vi "Dc_transparency_test_2.vi"() -> ()   [LabVIEW 2013]
uses:
  <vilib>/DAQmx/read.llb/DAQmx Read (Analog 1D DBL 1Chan NSamp).vi
  <vilib>/DAQmx/read.llb/DAQmx Read (Analog DBL 1Chan 1Samp).vi
  <vilib>/DAQmx/create/channels.llb/DAQmx Create Channel (AI-Voltage-Basic).vi
  <vilib>/DAQmx/configure/timing.llb/DAQmx Timing (Sample Clock).vi
  <vilib>/Utility/file.llb/Write To Spreadsheet File (DBL).vi
  <vilib>/DAQmx/miscellaneous.llb/DAQmx Fill In Error Info.vi
  <resource>/objmgr/daqmx.rc
panel:
  in  "Drop":dbl
  out "Waveform Chart 2":dbl[](graph)
  out "Measurement File":path=path "C:/Users/Adam/Desktop/Diag_Prog_v9/testt"
  out "Waveform Chart":dbl(graph)
  in  "Ref channel":tag="Dev3/ai2"
  in  "stop":bool
  in  "Timer Start":bool
  in  "Start time":timestamp=timestamp(-9593251199.274853 s since 1904-01-01)
  in  "Record Button":bool
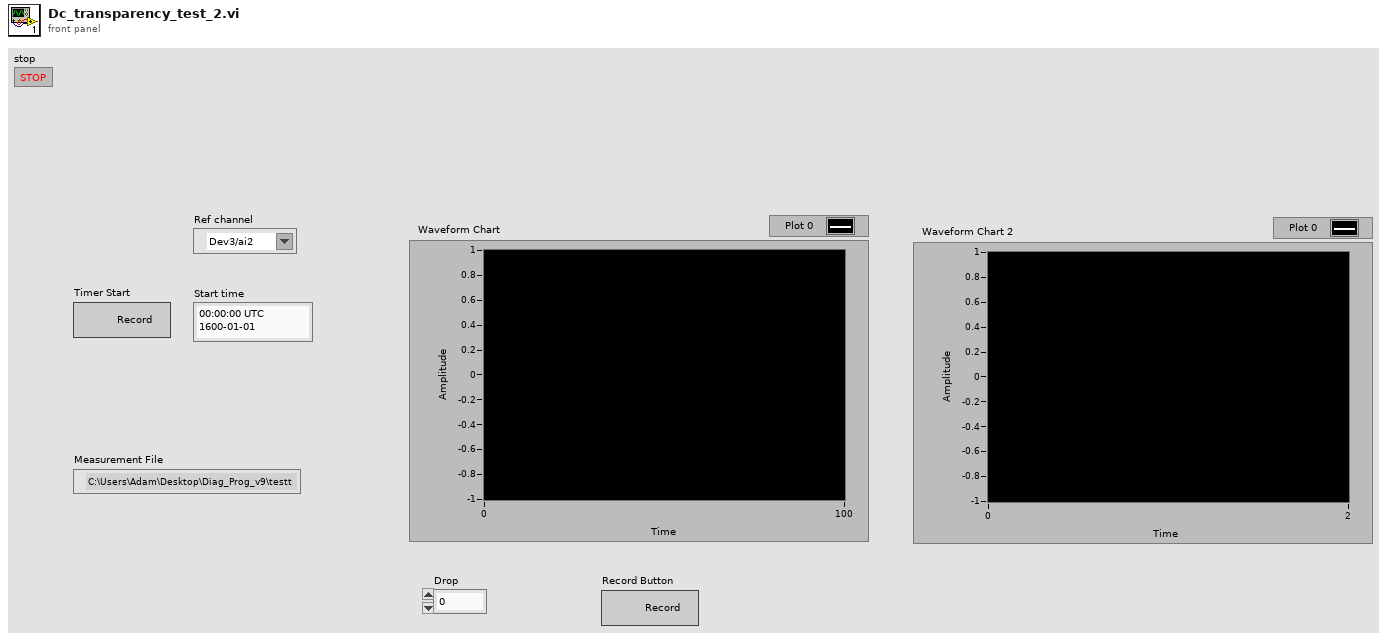
[diagram p1: front panel]
types:
  T1 = enum16{"open", "replace", "create", "open or create", "replace or create", "replace or create with confirmation"}
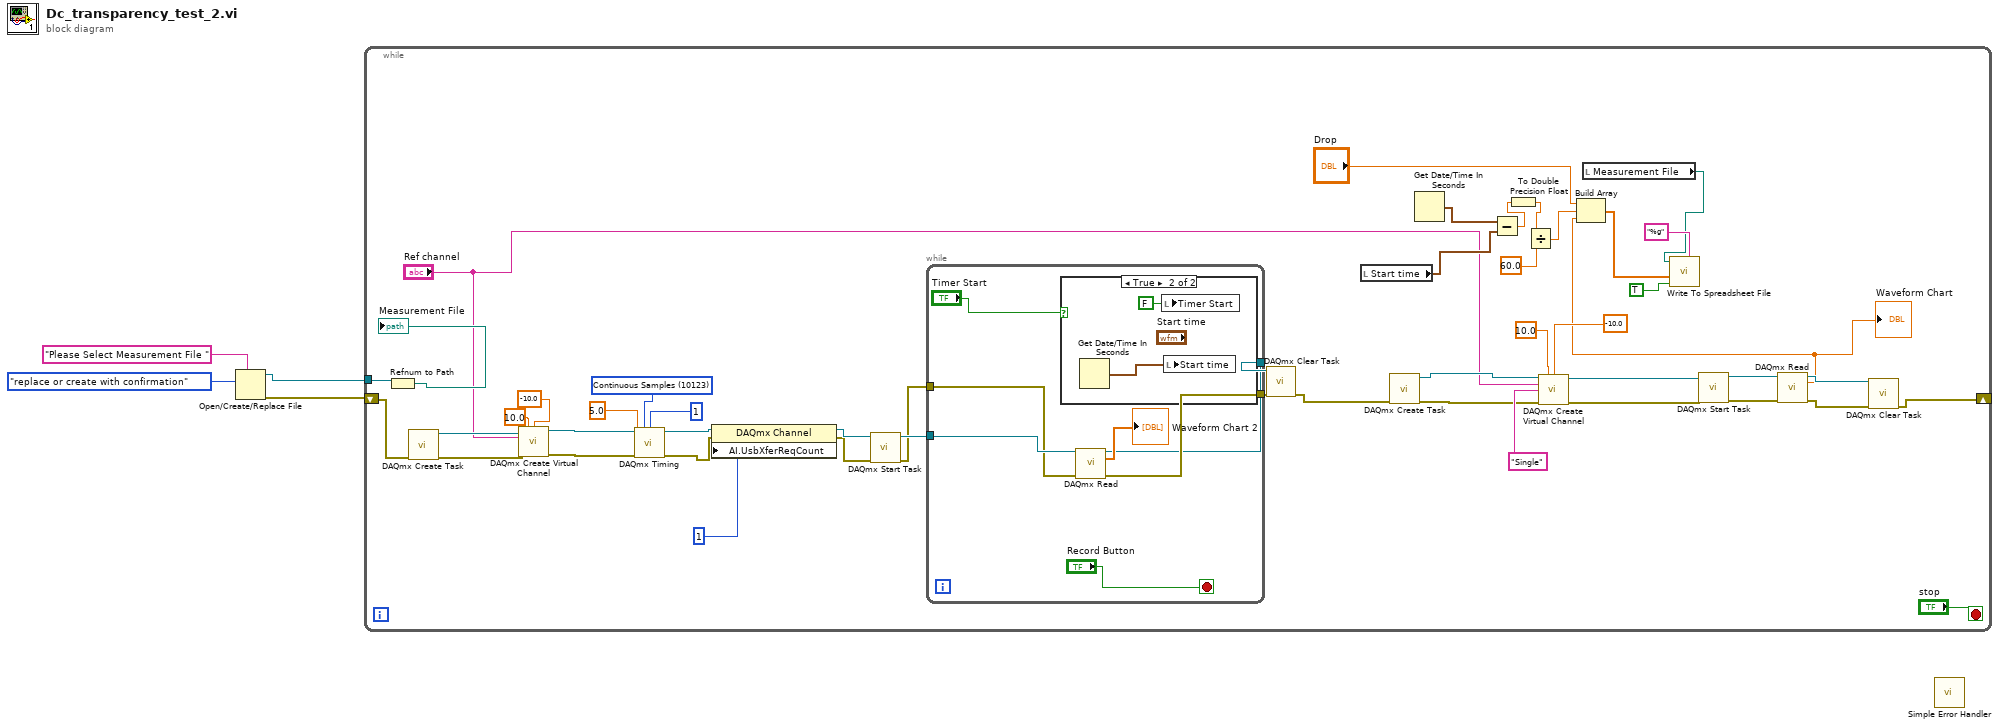
[diagram p0: block diagram]
diagram:
  n1 = Open/Create/Replace File(prompt="Please Select Measurement File ", operation (0:open)=T1."replace or create with confirmation") -> (refnum out=w2:refnum<file>, error out=w1:errorcluster)  [unwired: 4 in, 1 out]
  n2 = while {
    tunnel: w2 -> [w51]
    shift-right: [w12] -> _
    shift-left: w1 -> [w11]
    stop <- "stop" stop-if-true
    w15 = 10123 items=["Finite Samples"=10178, "Continuous Samples"=10123, "Hardware Timed Single Point"=12522] ("sample mode")
    n3 = Refnum to Path(1:w51) -> (0:→"Measurement File":path)
    n4 = call <vilib>:"DAQmx Create Task.vi"("error in"=w11) -> ("task out"=w14:refnum<k21>, "error out"=w13:errorcluster)  [unwired: 13 in]
    n5 = call-poly <vilib>:"DAQmx Create Virtual Channel.vi"("task in"=w14, "maximum value"=10.0, "minimum value"=-10.0, "physical channels"="Ref channel", "error in"=w13) -> ("task out"=w21:refnum<k21>, "error out"=w20:errorcluster)  [unwired: 9 in]
    n6 = call-poly <vilib>:"DAQmx Timing.vi"("task/channels in"=w21, "sample mode"=w15, "samples per channel"=1, "rate"=5.0, "error in"=w20) -> ("task out"=w16:refnum<k21>, "error out"=w17:errorcluster)  [unwired: 9 in]
    n7 = property class="DAQmx Channel"(reference=w16, error in=w17, "AI.UsbXferReqCount"=u32 1) -> (reference out=w10:refnum<k21>, error out=w9:errorcluster)
    n8 = call <vilib>:"DAQmx Start Task.vi"("task/channels in"=w10, "error in"=w9) -> ("task out"=w8:refnum<k21>, "error out"=w7:errorcluster)  [unwired: 12 in]
    n9 = while {
      tunnel: [w58] -> w49
      tunnel: [w56] -> w25
      tunnel: w8 -> [w55]
      tunnel: w7 -> [w54]
      stop <- "Record Button" stop-if-true
      n10 = case shown="True" "Timer Start" {
        frame False {
        }
        frame True {
          n11 = Get Date/Time In Seconds() -> (seconds since 1Jan1904=w61:timestamp)
          n12 = local write "Timer Start"(FALSE ("Timer Start")) -> ()
          n13 = local write "Start time"(w61) -> ()
        }
      }
      n14 = call-poly <vilib>:"DAQmx Read.vi"("task/channels in"=w55, "error in"=w54) -> ("task out"=w56:refnum<k21>, "data"=→"Waveform Chart 2":dbl[], "error out"=w58:errorcluster)  [unwired: 11 in]
    }
    n15 = call <vilib>:"DAQmx Clear Task.vi"("task in"=w25, "error in"=w49) -> ("error out"=w26:errorcluster)  [unwired: 13 in]
    n16 = local read "Start time"() -> (w30:timestamp)
    n17 = call <vilib>:"DAQmx Create Task.vi"("error in"=w26) -> ("task out"=w45:refnum<k21>, "error out"=w44:errorcluster)  [unwired: 13 in]
    n18 = Get Date/Time In Seconds() -> (seconds since 1Jan1904=w34:timestamp)
    n19 = Subtract(x=w34, y=w30) -> (x-y=w32:dbl)
    n20 = To Double Precision Float(number=w32) -> (double precision float=w31:dbl)
    n21 = Divide(x=w31, y=60.0) -> (x/y=w29:dbl)
    n22 = call-poly <vilib>:"DAQmx Create Virtual Channel.vi"("task in"=w45, "maximum value"=10.0, "minimum value"=-10.0, "physical channels"="Ref channel", "name to assign"="Single", "error in"=w44) -> ("task out"=w41:refnum<k21>, "error out"=w40:errorcluster)  [unwired: 8 in]
    n23 = local read "Measurement File"() -> (w27:path)
    n24 = call <vilib>:"DAQmx Start Task.vi"("task/channels in"=w41, "error in"=w40) -> ("task out"=w47:refnum<k21>, "error out"=w48:errorcluster)  [unwired: 12 in]
    n25 = call-poly <vilib>:"DAQmx Read.vi"("task/channels in"=w47, "error in"=w48) -> ("task out"=w38:refnum<k21>, "data"=w35:dbl, "error out"=w39:errorcluster)  [unwired: 11 in]
    "Waveform Chart" <- w35
    n26 = Build Array("Drop", w29, w35) -> (w28:dbl[])
    n27 = call-poly <vilib>:"Write To Spreadsheet File.vi"("format (%.3f)"="%g", "append to file? (new file:F)"=TRUE, "1D data"=w28, "file path (dialog if empty)"=w27) -> ()  [unwired: 4 in, 1 out]
    n28 = call <vilib>:"DAQmx Clear Task.vi"("task in"=w38, "error in"=w39) -> ("error out"=w12:errorcluster)  [unwired: 13 in]
  }
  n29 = call <vilib>:"Simple Error Handler.vi"() -> ()  [unwired: 5 in, 5 out]
